vi "user initialization.vi"(8 "error in":errorcluster, 10 "configuration in":refnum<class "control module configuration.lvclass">, 11 "fixed channel runtime in":refnum<class "control module runtime.lvclass">) -> (0 "error out":errorcluster, 3 "fixed channel runtime out":refnum<class "control module runtime.lvclass">)   [LabVIEW 2013, in "control module runtime.lvclass"]
uses:
  control module runtime.lvclass
  configuration/control module configuration.lvclass
  configuration/control module configuration.lvclass/control module configuration.ctl
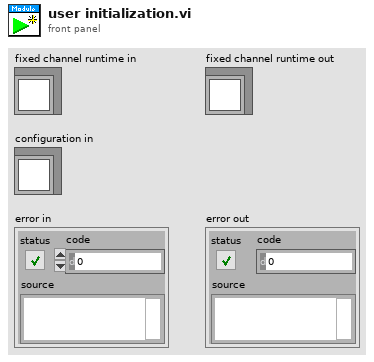
[diagram p1: front panel]
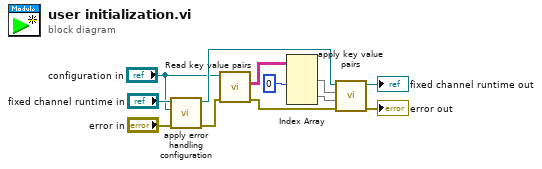
[diagram p0: block diagram]
diagram:
  n1 = call-dynamic "apply error handling configuration.vi"("error in"="error in", "configuration in"="configuration in", "fixed channel runtime in"="fixed channel runtime in") -> ("error out"=w4:errorcluster, "fixed channel runtime out"=w2:refnum<class "control module runtime.lvclass">)  [unwired: 7 in]
  n2 = call "Read key value pairs.vi"("error in"=w4, "fixed channel configuration in"="configuration in") -> ("error out"=w9:errorcluster, "key value pairs"=w12:string[][])  [unwired: 7 in, 1 out]
  n3 = Index Array(array=w12, index (col) #1=0 ("disabled index (col)")) -> (element #1=w7:string[], element #2=w6:string[])  [unwired: 3 in]
  n4 = call-dynamic "apply key value pairs.vi"("error in"=w9, "values"=w6, "keys"=w7, "fixed channel runtime in"=w2) -> ("error out"=→"error out":errorcluster, "fixed channel runtime out"=→"fixed channel runtime out":refnum<class "control module runtime.lvclass">)  [unwired: 6 in]
